vi "RealTimeMeasure2.vi"() -> ()   [LabVIEW 2012]
uses:
  <vilib>/Instr/_visa.llb/VISA Configure Serial Port (Instr).vi
panel:
  out "Vasak jalg hetkeväärtus":dbl
  out "Parem jalg hetkeväärtus":dbl
  out "Parem jalg":cluster{timestamp[], dbl[]}(graph)
  out "Vasak jalg":cluster{timestamp[], dbl[]}(graph)
  in  "Numeric":i32=20
  in  "stop":bool
  in  "VISA Refnum in":refnum<visa-resource-name>="COM1"
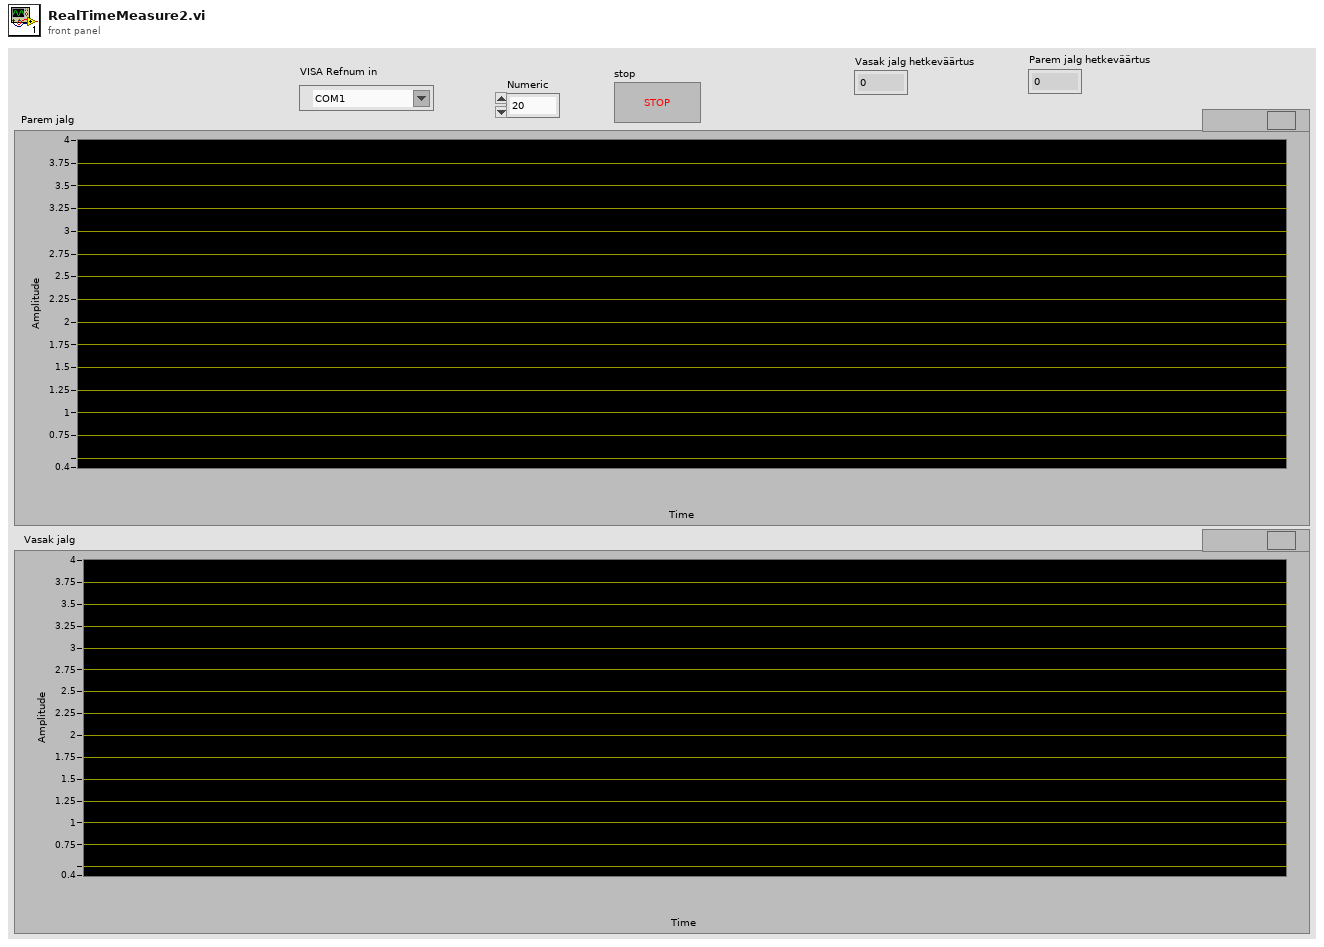
[diagram p1: front panel]
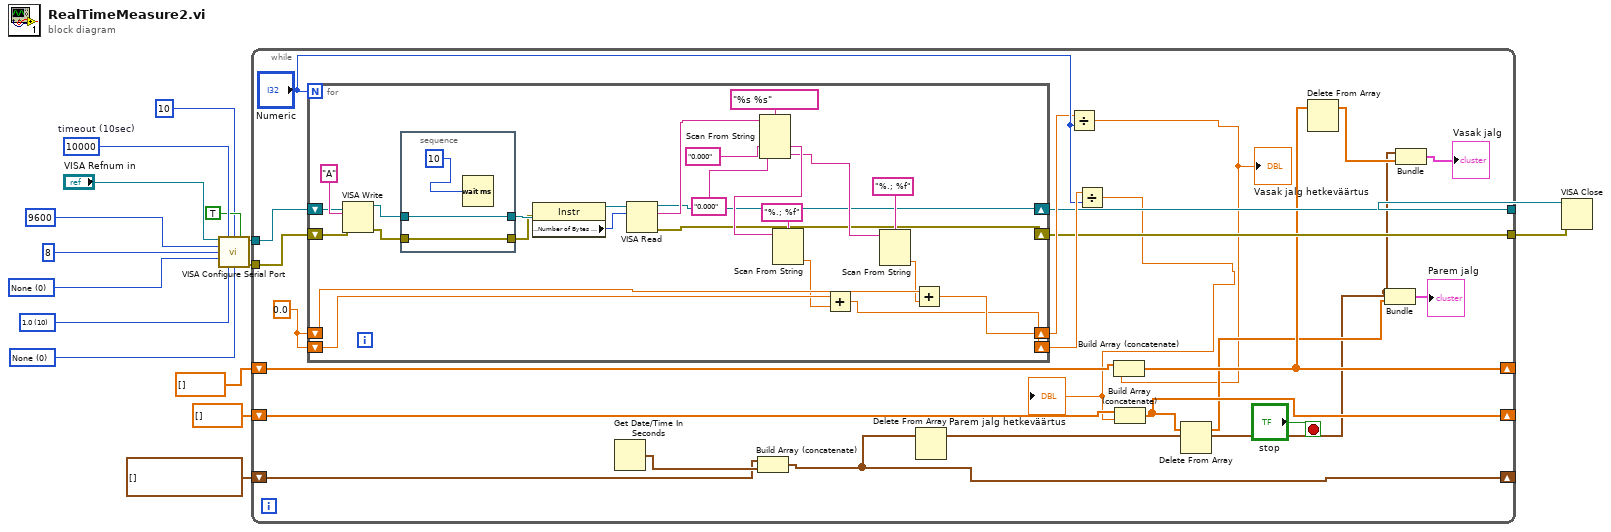
[diagram p0: block diagram]
diagram:
  w16 = u16 0 items=["None"=0, "XON/XOFF"=1, "RTS/CTS"=2, "DTR/DSR"=4] ("flow control")
  w15 = u16 10 items=["1.0"=10, "1.5"=15, "2.0"=20] ("stop bits")
  w14 = u16 0 items=["None", "Odd", "Even", "Mark", "Space"] ("parity")
  w10 = u32 10000  # timeout (10sec)
  n1 = call-poly "VISA Configure Serial Port"("VISA resource name"="VISA Refnum in", "timeout (10sec)"=w10, "termination char\n(0xA = '\\n' = LF)"=u8 10 ("termination char\n(0xA = '\\n' = LF)"), "Enable Termination\nChar (T)"=TRUE ("Enable Termination\nChar (T)"), "baud rate (9600)"=u32 9600 ("baud rate"), "data bits (8)"=u16 8 ("data bits"), "parity (0:none)"=w14, "stop bits (10: 1 bit)"=w15, "flow control (0:none)"=w16) -> ("VISA resource name out"=w9:refnum<visa-resource-name>, "error out"=w8:errorcluster)  [unwired: 1 in, 4 out]
  n2 = while {
    tunnel: w9 -> [w38]
    tunnel: w8 -> [w31]
    shift-right: [w24] -> _
    shift-left: dbl[] [] -> [w34]
    shift-right: [w19] -> _
    shift-left: timestamp[] [] -> [w32]
    tunnel: [w29] -> w4
    tunnel: [w28] -> w3
    shift-right: [w26] -> _
    shift-left: dbl[] [] -> [w27]
    stop <- "stop" stop-if-true
    w37 = 0.0 ("x")
    n3 = for {
      N: "Numeric" -> [_]
      shift-right: [w49] -> w29
      shift-left: w38 -> [w47]
      shift-right: [w48] -> w28
      shift-left: w31 -> [w46]
      shift-right: [w40] -> w36
      shift-left: w37 -> [w45]
      shift-right: [w41] -> w30
      shift-left: w37 -> [w44]
      n4 = VISA Write(VISA resource name=w47, write buffer="A" ("Command String"), error in (no error)=w46) -> (VISA resource name out=w63:refnum<visa-resource-name>, error out=w62:errorcluster)  [unwired: 1 out]
      n5 = stacked-sequence {
        tunnel: w62 -> [w67]
        tunnel: [w67] -> w58
        tunnel: w63 -> [w66]
        tunnel: [w66] -> w59
        frame #0 {
          n6 = Wait (ms)(milliseconds to wait=u32 10 ("delay Command")) -> ()  [unwired: 1 out]
        }
      }
      n7 = property class="Instr"(reference=w59, error in=w58) -> (reference out=w61:refnum<visa-resource-name>, "Serial Settings:Number of Bytes at Serial Port"=w60:u32)  [unwired: 1 out]
      n8 = VISA Read(VISA resource name=w61, byte count=w60) -> (VISA resource name out=w49:refnum<visa-resource-name>, read buffer=w57:string, error out=w48:errorcluster)  [unwired: 1 in, 1 out]
      n9 = Scan From String(format string="%s %s", input string=w57, default 1="0.000", default 2="0.000") -> (output 1=w51:string, output 2=w50:string)  [unwired: 2 in, 3 out]
      n10 = Scan From String(format string="%.; %f", input string=w51) -> (output 1=w43:dbl)  [unwired: 3 in, 3 out]
      n11 = Add(x=w45, y=w43) -> (x+y=w40:dbl)
      n12 = Scan From String(format string="%.; %f", input string=w50) -> (output 1=w42:dbl)  [unwired: 3 in, 3 out]
      n13 = Add(x=w44, y=w42) -> (x+y=w41:dbl)
    }
    n14 = Get Date/Time In Seconds() -> (seconds since 1Jan1904=w33:timestamp)
    n15 = Build Array (concatenate)(w32, w33) -> (w19:timestamp[])
    n16 = Delete From Array(array=w19) -> (array with subset deleted=w22:timestamp[])  [unwired: 2 in, 1 out]
    n17 = Divide(x=w30, y="Numeric") -> (x/y=w18:dbl)
    "Vasak jalg hetkeväärtus" <- w18
    n18 = Divide(x=w36, y="Numeric") -> (x/y=w17:dbl)
    "Parem jalg hetkeväärtus" <- w17
    n19 = Build Array (concatenate)(w27, w18) -> (w26:dbl[])
    n20 = Build Array (concatenate)(w34, w17) -> (w24:dbl[])
    n21 = Delete From Array(array=w24) -> (array with subset deleted=w23:dbl[])  [unwired: 2 in, 1 out]
    n22 = Delete From Array(array=w26) -> (array with subset deleted=w25:dbl[])  [unwired: 2 in, 1 out]
    n23 = Bundle(w22, w23) -> (→"Parem jalg":cluster{timestamp[], dbl[]})  [unwired: 1 in]
    n24 = Bundle(w22, w25) -> (→"Vasak jalg":cluster{timestamp[], dbl[]})  [unwired: 1 in]
  }
  n25 = VISA Close(VISA resource name=w4, error in (no error)=w3) -> ()  [unwired: 1 out]
